vi "getArrayLength.vi"(4 "error in":errorcluster, 7 "msg in":string) -> (0 "error out":errorcluster, 2 "array length":u32, 3 "msg out":string)   [LabVIEW 2012]
doc: "Parses out an array length from msg in. Returns the rest of string in msg out.\n\nUseful for parsing variable length arrays of non-primitive types. See parse_point_cloud.vi for usage example."
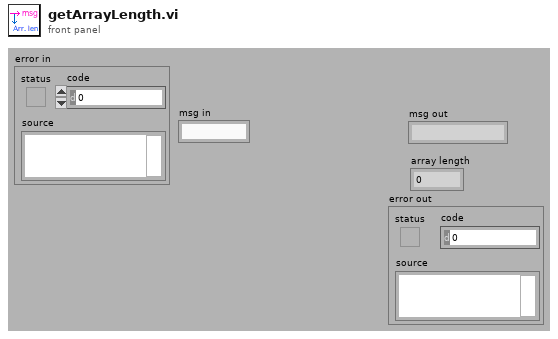
[diagram p1: front panel]
types:
  T1 = enum16{"big-endian, network order", "native, host order", "little-endian"}
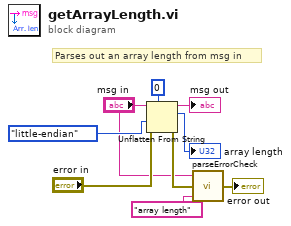
[diagram p0: block diagram]
diagram:
  # "Parses out an array length from msg in"
  n1 = Unflatten From String(type=u32 0, binary string="msg in", byte order (0:big-endian, network order)=T1."little-endian", error in (no error)="error in") -> (rest of the binary string=→"msg out":string, value=→"array length":u32, error out=w4:errorcluster)  [unwired: 1 in]
  n2 = call "parseErrorCheck.vi"("type"="array length", "error in"=w4, "msg read"="msg in") -> ("error out"=→"error out":errorcluster)
